vi "Close.vi"(8 "error in (no error)":errorcluster, 11 "NI DMM4072 in":refnum<class "NI DMM4072.lvclass">) -> (0 "error out":errorcluster, 3 "NI DMM4072 out":refnum<class "NI DMM4072.lvclass">)   [LabVIEW 2019, in "Concrete.lvlib" / "NI DMM4072.lvclass"]
uses:
  NI DMM4072.lvclass
  NI DMM4072.lvclass/NI DMM4072.ctl
  Harware Abstraction/MultiIO/MIO.lvclass
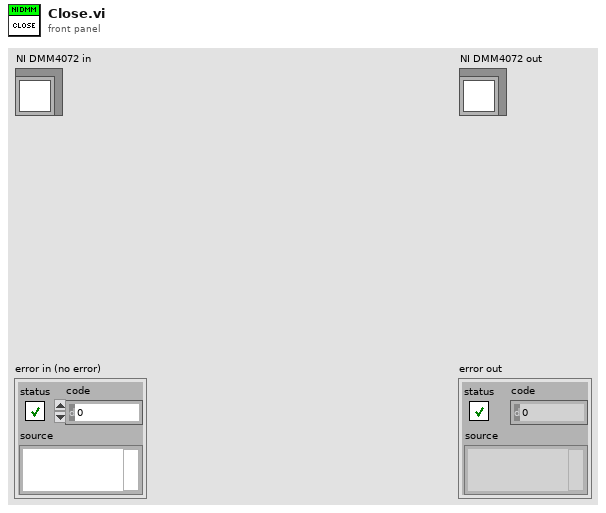
[diagram p1: front panel]
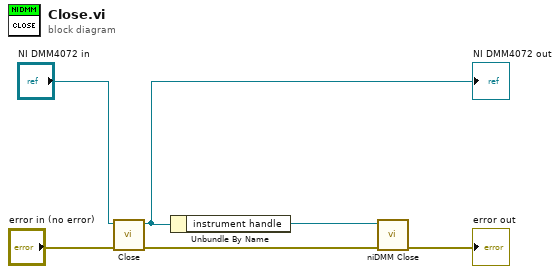
[diagram p0: block diagram]
diagram:
  n1 = call-parent "Close.vi"("error in (no error)"="error in (no error)", "Instrument in"="NI DMM4072 in") -> ("error out"=w2:errorcluster, "Instrument out"=w4:refnum<class "NI DMM4072.lvclass">)  [unwired: 8 in]
  "NI DMM4072 out" <- w4
  n2 = Unbundle By Name(w4) -> ("instrument handle"=w3:refnum<k15>)
  n3 = call <instrlib>:"niDMM Close.vi"("error in (no error)"=w2, "instrument handle"=w3) -> ("error out"=→"error out":errorcluster)  [unwired: 9 in]
